vi "Format Help Path String.vi"(11 "Help Path":path) -> (3 "Help Path String":string)   [LabVIEW 2020, in "VI Properties Editor.lvlib"]
doc: "Formats <B>Help Path</B> into a string to be displayed, outputting an empty string if it is <Not A Path>."
uses:
  VI Properties Editor.lvlib
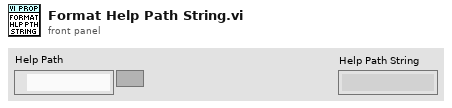
[diagram p1: front panel]
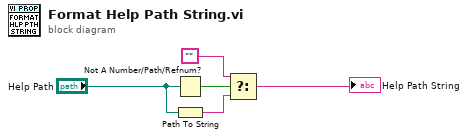
[diagram p0: block diagram]
diagram:
  n1 = Not A Number/Path/Refnum?(number/path/refnum="Help Path") -> (NaN/Path/Refnum?=w3:bool)
  n2 = Path To String(path="Help Path") -> (string=w2:string)
  n3 = Select(t="", s=w3, f=w2) -> (s? t:f=→"Help Path String":string)
